vi "CALCOLO NPSH.vi"(8 "H1":dbl, 9 "Ec1":dbl, 10 "Hv":dbl, 11 "Hbar":dbl) -> (3 "NPSH":dbl)   [LabVIEW 2019]
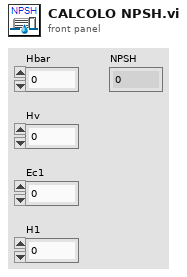
[diagram p1: front panel]
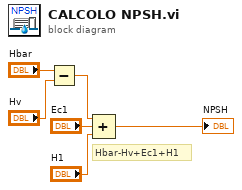
[diagram p0: block diagram]
diagram:
  # "Hbar-Hv+Ec1+H1"
  n1 = Subtract(x="Hbar", y="Hv") -> (x-y=w4:dbl)
  n2 = Compound Arithmetic op=ADD(w4, "Ec1", "H1") -> (→"NPSH":dbl)
